vi "parse_response.vi"(8 "error in":errorcluster, 11 "Response":string) -> (0 "error out":errorcluster, 2 "Meta Data":T1)   [LabVIEW 2020, in "Nominal Client.lvclass"]
uses:
  Nominal Client/Nominal Client.lvclass
  Nominal Client/Nominal Client.lvclass/Nominal Client.ctl
  bcb0b382-5e64-4907-9ede-aec9321e7f5a.vi
  metadata.ctl
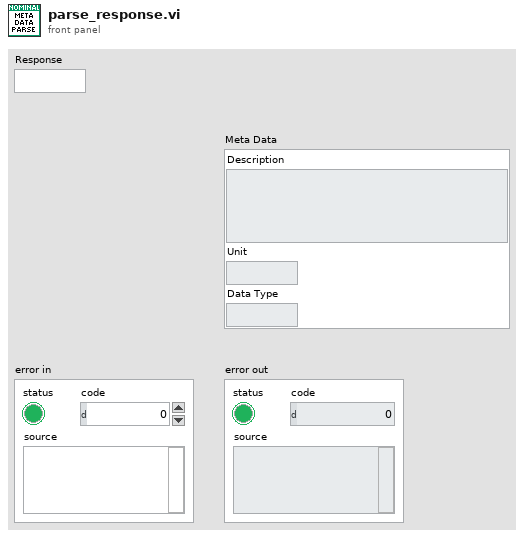
[diagram p1: front panel]
types:
  T1 = typedef "Nominal Client.lvclass/metadata.ctl" = cluster{"Description":string, "Unit":string, "Data Type":string}
  T2 = cluster{"[0]":string, "[1]":string, "[2]":string}
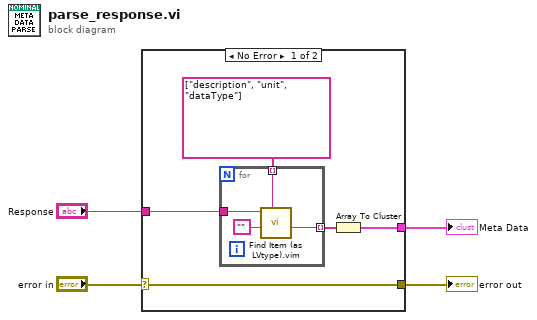
[diagram p0: block diagram]
diagram:
  n1 = case shown="No Error" "error in" {
    selector: "error in" -> [w5 w14]
    tunnel: "Response" -> [w9 _]
    tunnel: [w6 _] -> w3
    tunnel: [w5 w14] -> w1
    frame No Error {
      n2 = for {
        tunnel: w9 -> [w13]
        tunnel: string[] ["description", "unit", "dataType"] -> [w12] mode=indexing
        tunnel: [w10] -> w7 mode=indexing
        n3 = call "Find Item (as LVtype).vim"("$Path or Item Name"=w12, "Data Type and Default Value"="", "JSON"=w13) -> ("Data"=w10:string)  [unwired: 5 in, 3 out]
      }
      n4 = Array To Cluster(array=w7) -> (cluster=w6:T2)
    }
    frame Error {
    }
  }
  "Meta Data" <- w3
  "error out" <- w1
